vi "Check if Has Events.vi"(8 "error in (no error)":errorcluster, 11 "JKI SM in":refnum<class "JKI SM.lvclass">) -> (0 "error out":errorcluster, 2 "Has Dyanamic Events?":bool, 3 "JKI SM out":refnum<class "JKI SM.lvclass">)   [LabVIEW 2020, in "JKI State Machine API.lvlib" / "JKI SM.lvclass"]
uses:
  JKI SM.lvclass
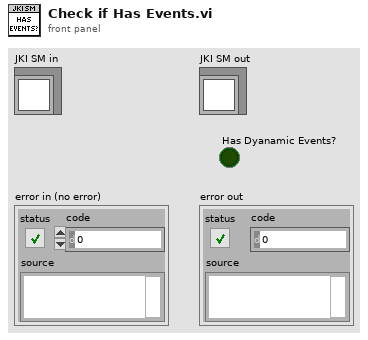
[diagram p1: front panel]
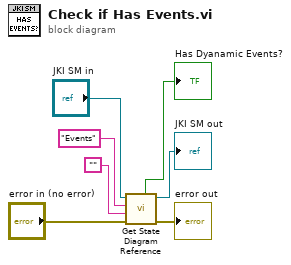
[diagram p0: block diagram]
diagram:
  n1 = call "Get State Diagram Reference.vi"("error in (no error)"="error in (no error)", "State Name"="", "Category (Optional)"="Events", "JKI SM in"="JKI SM in") -> ("error out"=→"error out":errorcluster, "JKI SM out"=→"JKI SM out":refnum<class "JKI SM.lvclass">, "Found?"=→"Has Dyanamic Events?":bool)  [unwired: 3 in, 2 out]
